vi "4.3.vi"() -> ()   [LabVIEW 2017]
panel:
  out "Y":dbl
  out "X":dbl
  in  "数值":dbl
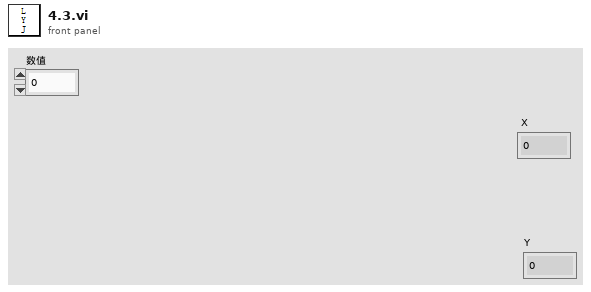
[diagram p1: front panel]
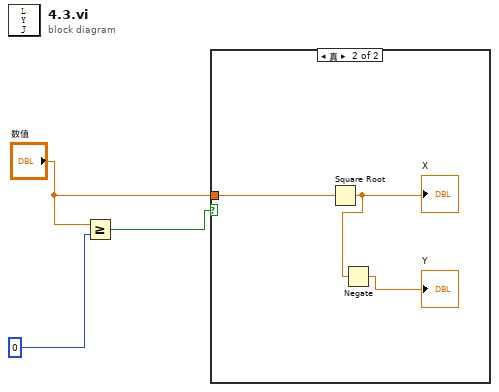
[diagram p0: block diagram]
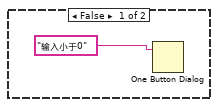
[diagram p2: hidden frame]
diagram:
  n1 = Greater Or Equal?(x="数值", y=0) -> (x >= y?=w2:bool)
  n2 = case shown="真" w2 {
    tunnel: "数值" -> [_ w7]
    frame False {
      n3 = One Button Dialog(message="输入小于0") -> ()  [unwired: 1 in, 1 out]
    }
    frame True {
      n4 = Square Root(x=w7) -> (sqrt(x)=w6:dbl)
      "X" <- w6
      n5 = Negate(x=w6) -> (-x=→"Y":dbl)
    }
  }
